vi "ScreenShots_independent_VIs.vi"(8 "error in":errorcluster, 9 "referenz":refnum<vi>[](array[refnum]), 10 "filename":string[](array[string]), 11 "Screenshots Pfad":path) -> (0 "error out":errorcluster, 3 "Screenshots Pfad  out":path caption="Screenshots Pfad")   [LabVIEW 2020, in "Backup.lvlib"]
uses:
  Backup.lvlib
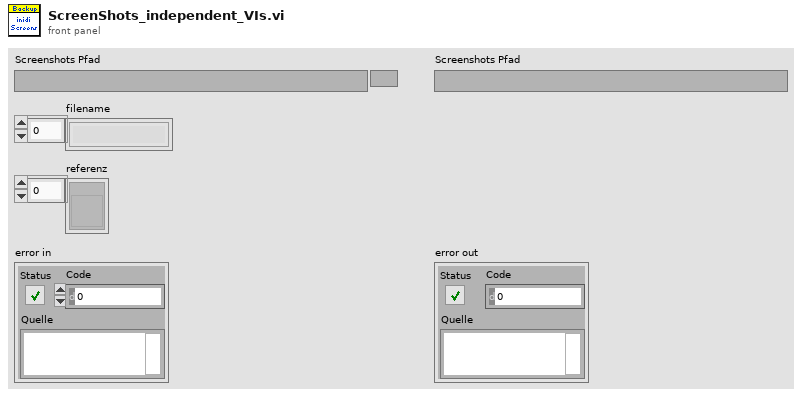
[diagram p1: front panel]
types:
  T1 = enum32{"Bad", "Idle", "Run top level", "Running"}
  T2 = typedef "imagedata.ctl" = cluster{"image type":i32, "image depth":i32, "image":u8[], "mask":u8[], "colors":u32[], "Rectangle":cluster{"left":i16, "top":i16, "right":i16, "bottom":i16}}
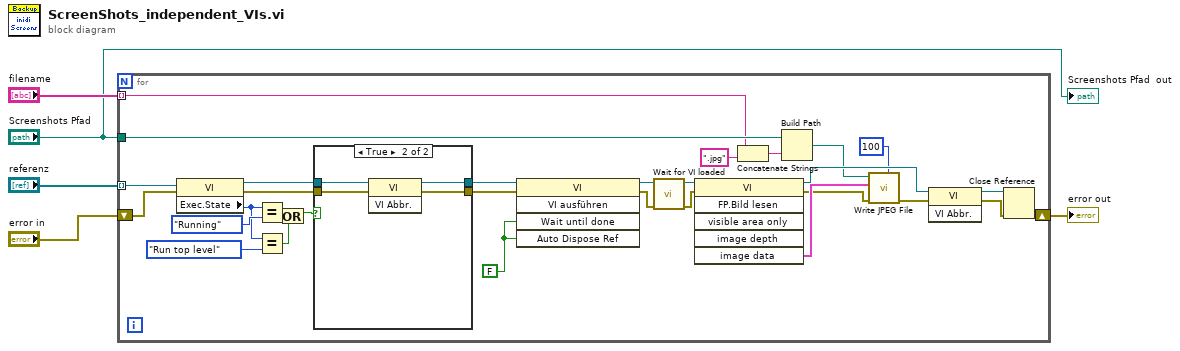
[diagram p0: block diagram]
diagram:
  n1 = for {
    tunnel: "Screenshots Pfad" -> [w35]
    tunnel: "referenz" -> [w17] mode=indexing
    tunnel: "filename" -> [w10] mode=indexing
    shift-right: [w30] -> w5
    shift-left: "error in" -> [w28]
    w27 = FALSE
    n2 = property class="VI"(reference=w17, error in=w28) -> (reference out=w26:refnum<vi>, error out=w23:errorcluster, "Exec.State"=w20:T1)
    n3 = Equal?(x=w20, y=T1."Running" ("Ausführung:Status")) -> (x = y?=w24:bool)
    n4 = Equal?(x=w20, y=T1."Run top level" ("Ausführung:Status")) -> (x = y?=w18:bool)
    n5 = Or(x=w24, y=w18) -> (x .or. y?=w19:bool)
    n6 = case shown="True" w19 {
      tunnel: w26 -> [w37 w41]
      tunnel: [w37 w40] -> w25
      tunnel: w23 -> [w36 w39]
      tunnel: [w36 w38] -> w22
      frame False {
      }
      frame True {
        n7 = invoke class="VI" method="VI Abbr."(reference=w41, error in=w39) -> (reference out=w40:refnum<vi>, error out=w38:errorcluster)  [unwired: 1 in, 1 out]
      }
    }
    n8 = invoke class="VI" method="VI ausführen"(reference=w25, error in=w22, "Wait until done"=w27, "Auto Dispose Ref"=w27) -> (reference out=w9:refnum<vi>, error out=w7:errorcluster)  [unwired: 1 in, 3 out]
    n9 = call "Wait for VI loaded.vi"("error in"=w7, "VI Referenz"=w9) -> ("error out"=w6:errorcluster, "VI Referenz out"=w8:refnum<vi>)  [unwired: 7 in, 1 out]
    n10 = invoke class="VI" method="FP.Bild lesen"(reference=w8, error in=w6) -> (reference out=w33:refnum<vi>, error out=w15:errorcluster, "image data"=w16:T2)  [unwired: 4 in, 3 out]
    n11 = Concatenate Strings(w10, ".jpg" ("String")) -> (w12:string)
    n12 = Build Path(base path=w35, name or relative path=w12) -> (appended path=w13:path)
    n13 = call <vilib>:"Write JPEG File.vi"("quality (80)"=100, "error in (no error)"=w15, "image data"=w16, "path to JPEG file"=w13) -> ("error out"=w34:errorcluster)  [unwired: 6 in, 1 out]
    n14 = invoke class="VI" method="VI Abbr."(reference=w33, error in=w34) -> (reference out=w32:refnum<vi>, error out=w31:errorcluster)  [unwired: 1 in, 1 out]
    n15 = Close Reference(reference=w32, error in (no error)=w31) -> (error out=w30:errorcluster)
  }
  "error out" <- w5
  "Screenshots Pfad  out" <- "Screenshots Pfad"
